vi "FormatVoltageArray_V2.vi"(11 "Array in":dbl[](array[numeric])) -> (0 "Mirror Array":u16[](array[numeric]), 3 "Voltage Map":dbl[][](array[numeric]))   [LabVIEW 2015]
uses:
  <vilib>/Analysis/baseanly.llb/Mean (DBL).vi
  <vilib>/Analysis/NI_AALBase.lvlib
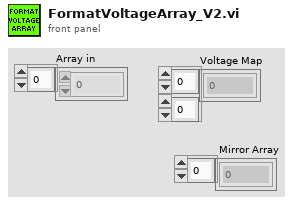
[diagram p1: front panel]
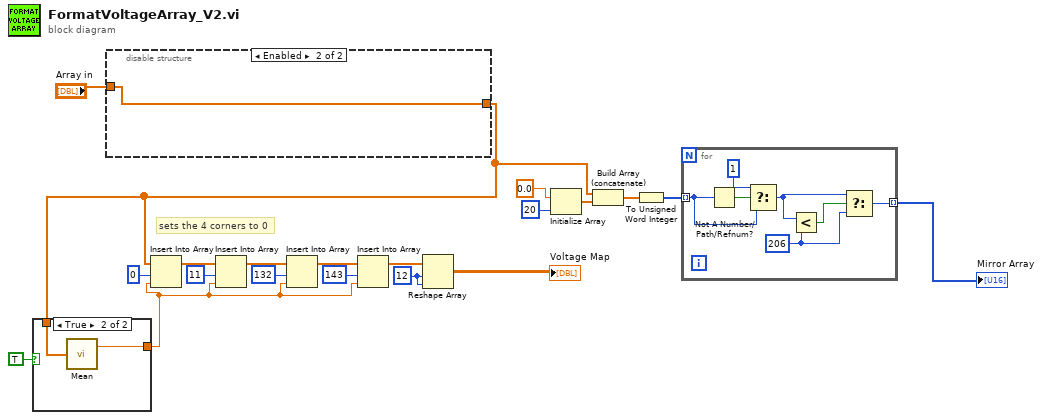
[diagram p0: block diagram]
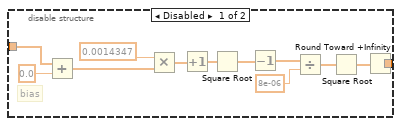
[diagram p2: hidden frame]
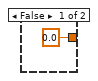
[diagram p3: hidden frame]
diagram:
  w12 = 12 ("dimension size")
  # "sets the 4 corners to 0"
  n1 = disable-structure shown="Enabled" {
    disable-tunnel: "Array in" -> [w32 w33]
    disable-tunnel: [w31 w33] -> w3
    frame Disabled {
      # "bias"
      n2 = Add(x=w32, y=0.0) -> (x+y=w27:dbl[])
      n3 = Multiply(x=0.0014347, y=w27) -> (x*y=w26:dbl[])
      n4 = Increment(x=w26) -> (x+1=w25:dbl[])
      n5 = Square Root(x=w25) -> (sqrt(x)=w24:dbl[])
      n6 = Decrement(x=w24) -> (x-1=w22:dbl[])
      n7 = Divide(x=w22, y=8e-06) -> (x/y=w21:dbl[])
      n8 = Square Root(x=w21) -> (sqrt(x)=w30:dbl[])
      n9 = Round Toward +Infinity(x=w30) -> (ceil(x): smallest int >= x=w31:dbl[])
    }
    frame Enabled {
    }
  }
  n10 = case shown="True" TRUE {
    tunnel: w3 -> [_ w36]
    tunnel: [0.0 ("mean") w35] -> w2
    frame False {
    }
    frame True {
      n11 = call-poly <vilib>:"Mean.vi"("X"=w36) -> ("mean"=w35:dbl)  [unwired: 1 out]
    }
  }
  n12 = Insert Into Array(array=w3, index=0, new element=w2) -> (w17:dbl[])
  n13 = Insert Into Array(array=w17, index=11, new element=w2) -> (w15:dbl[])
  n14 = Insert Into Array(array=w15, index=132, new element=w2) -> (w13:dbl[])
  n15 = Insert Into Array(array=w13, index=143, new element=w2) -> (w11:dbl[])
  n16 = Reshape Array "Reshape Array"(w11, w12, w12) -> (→"Voltage Map":dbl[][])
  n17 = Initialize Array(0.0 ("element"), 20 ("dimension size")) -> (w9:dbl[])
  n18 = Build Array (concatenate)(w3, w9) -> (w6:dbl[])
  n19 = To Unsigned Word Integer(number=w6) -> (unsigned 16bit integer=w5:u16[])
  n20 = for {
    tunnel: w5 -> [w42] mode=indexing
    tunnel: [w37] -> w4 mode=indexing
    w38 = u16 206 ("y")
    n21 = Not A Number/Path/Refnum?(number/path/refnum=w42) -> (NaN/Path/Refnum?=w43:bool)
    n22 = Select(t=u16 1, s=w43, f=w42) -> (s? t:f=w39:u16)
    n23 = Less?(x=w39, y=w38) -> (x < y?=w40:bool)
    n24 = Select(t=w39, s=w40, f=w38) -> (s? t:f=w37:u16)
  }
  "Mirror Array" <- w4
